vi "放射性半衰期.vi"() -> ()   [LabVIEW 2014]
uses:
  <vilib>/Utility/file.llb/Write To Spreadsheet File (DBL).vi
panel:
  out "m":dbl
  out "每个数据的起始时间":u32
  out "是否为本底":bool
  in  "初始计数率":u32=5000 max=2000000
  out "设置：测量步长":dbl
  out "设置：测量时间":dbl
  out "时间缓存数组":dbl[](array[numeric])
  out "计数缓存数组":dbl[](array[numeric])
  out "图像缓存数组":dbl[][](array[numeric])
  out "n":dbl
  out "现在时间":u32
  in  "按钮_提示":bool caption="提示"
  in  "单道道宽":dbl
  in  "单道阈值":dbl
  out "测量状态":bool
  in  "选项卡控件_实验原理":enum32{"选项卡 1", "选项卡 2"}(tab)
  in  "选项卡控件 实验步骤":enum32{"选项卡 1", "选项卡 2"}(tab)
  in  "按钮_设置成本底":bool
  in  "按钮_保存":bool
  in  "时间步长":dbl caption="秒"
  in  "按钮_设置测量时间":bool
  in  "测量时间":dbl caption="秒"
  out "XY图":T1(graph)
  out "单道计数":i32
  out "停止变量":bool
  in  "按钮_退出":bool
  in  "按钮_开始测量":bool
  in  "按钮_停止":bool
  out "退出":bool
  # "实验：放射性半衰期"
  # "实验仪器"
  # "实验原理"
  # "实验步骤"
  # "操作面板"
  # "1.连接好仪器，放置活性化样品116mIn；\n      2.设置测量时间和测量时间步长；\n      3.点击开始测量，观察计数随着时间增加有着怎样的变化规律，图中的每个点代表每个步长时间间隔内的总计数；\n      4.当测量完成后，点击保存，选择路径并输入文件名；\n      5.点击设置成本底，测量本底10分钟；"
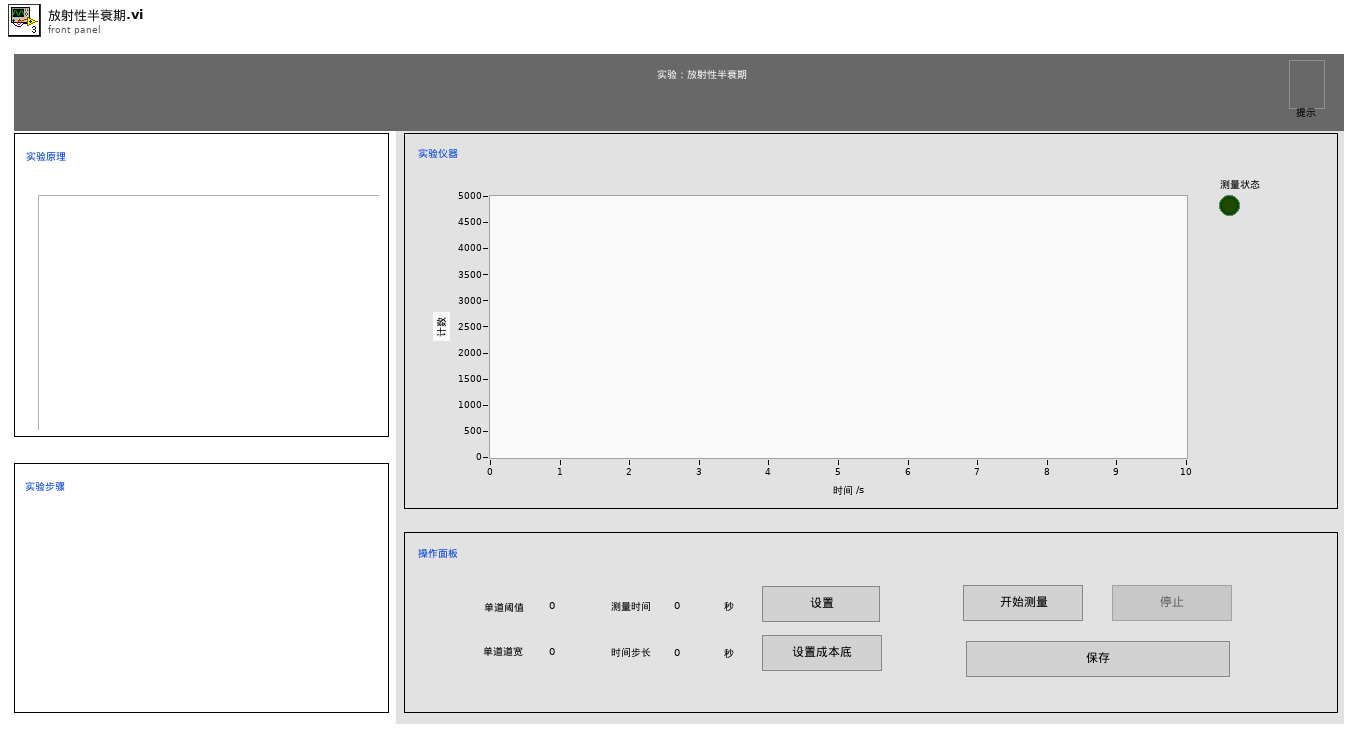
[diagram p1: front panel]
types:
  T1 = cluster{"表一：峰位——能量关系曲线图":cluster{"String":dbl, "String":dbl}[]}[]
  T2 = enum8{"Enabled", "Disabled", "Disabled and Grayed Out"}
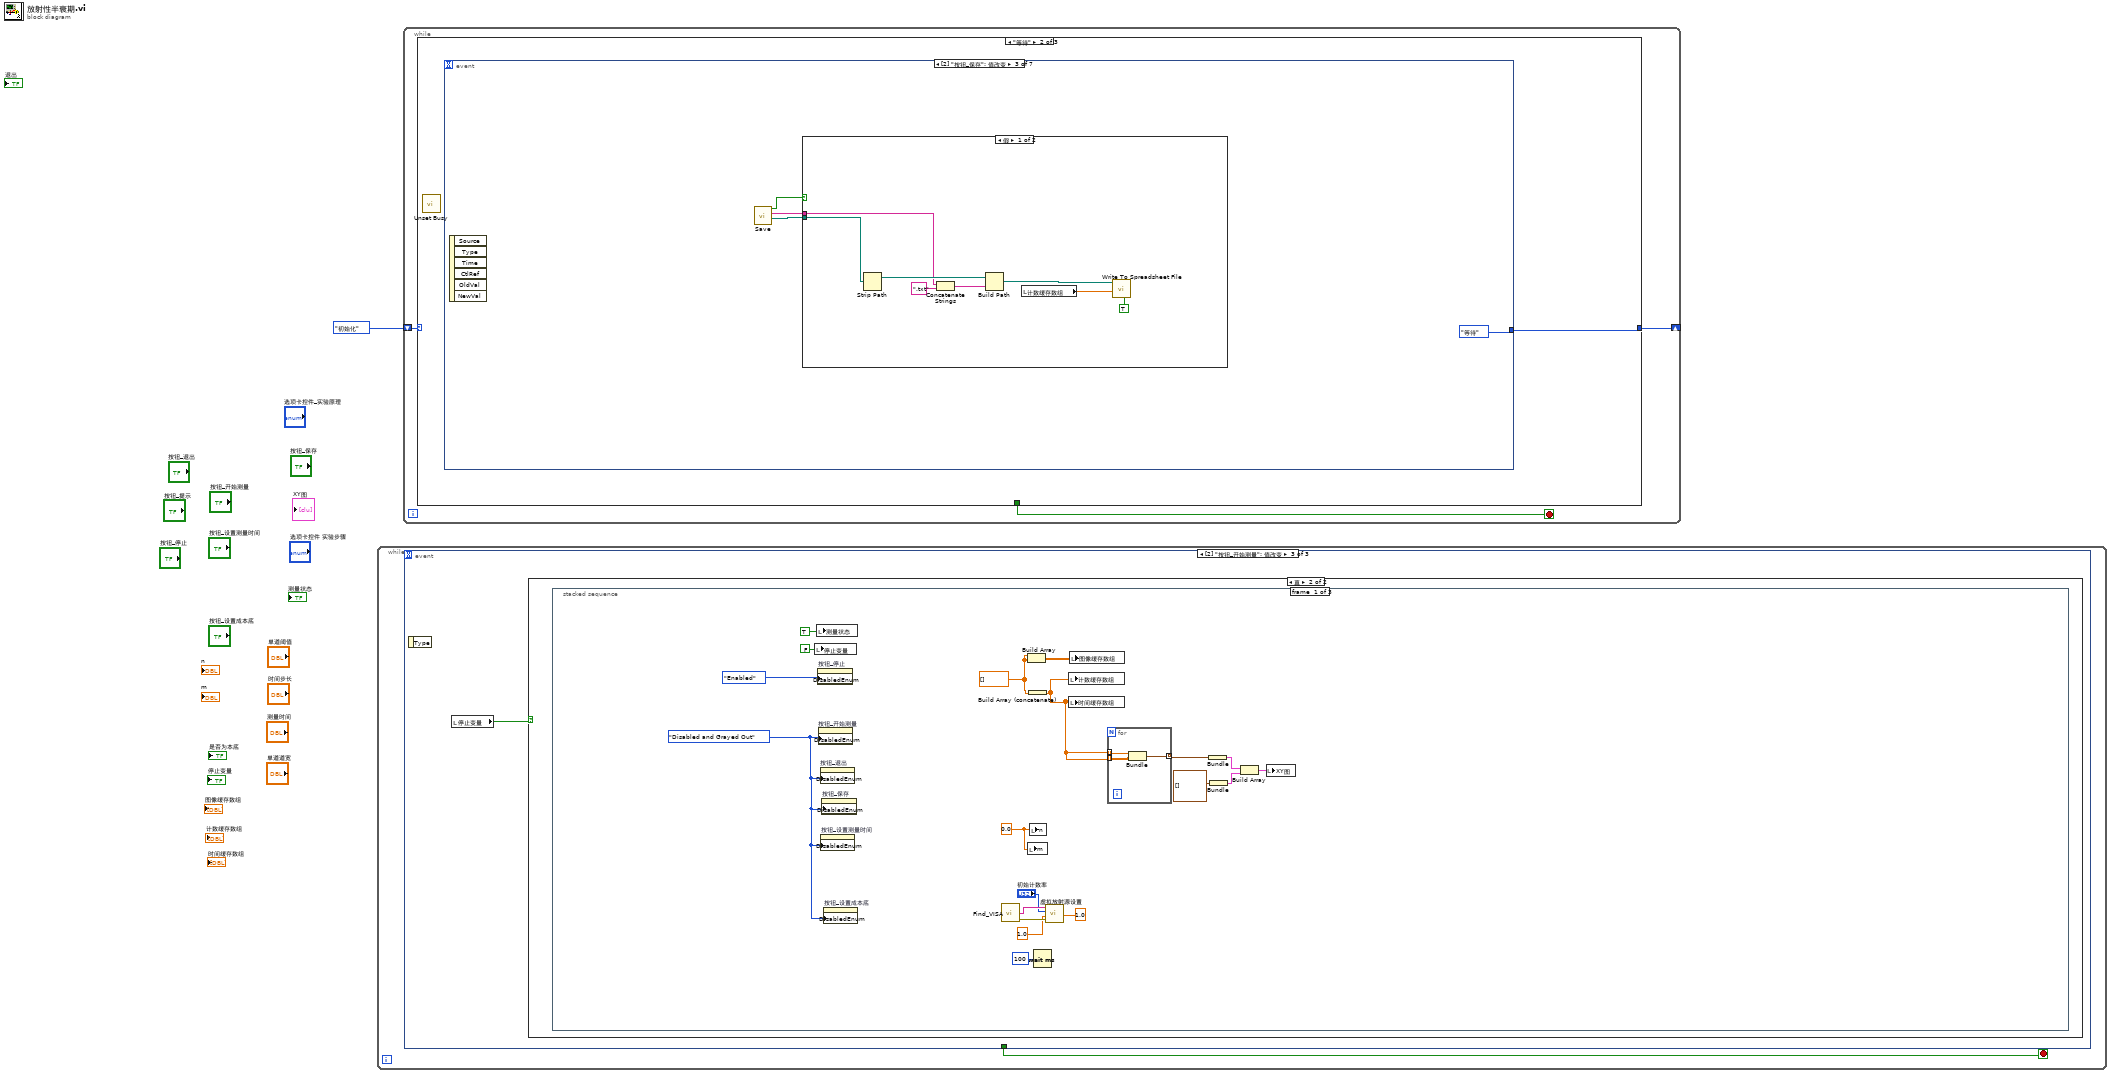
[diagram p0: block diagram]
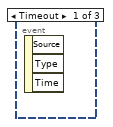
[diagram p2: hidden frame]
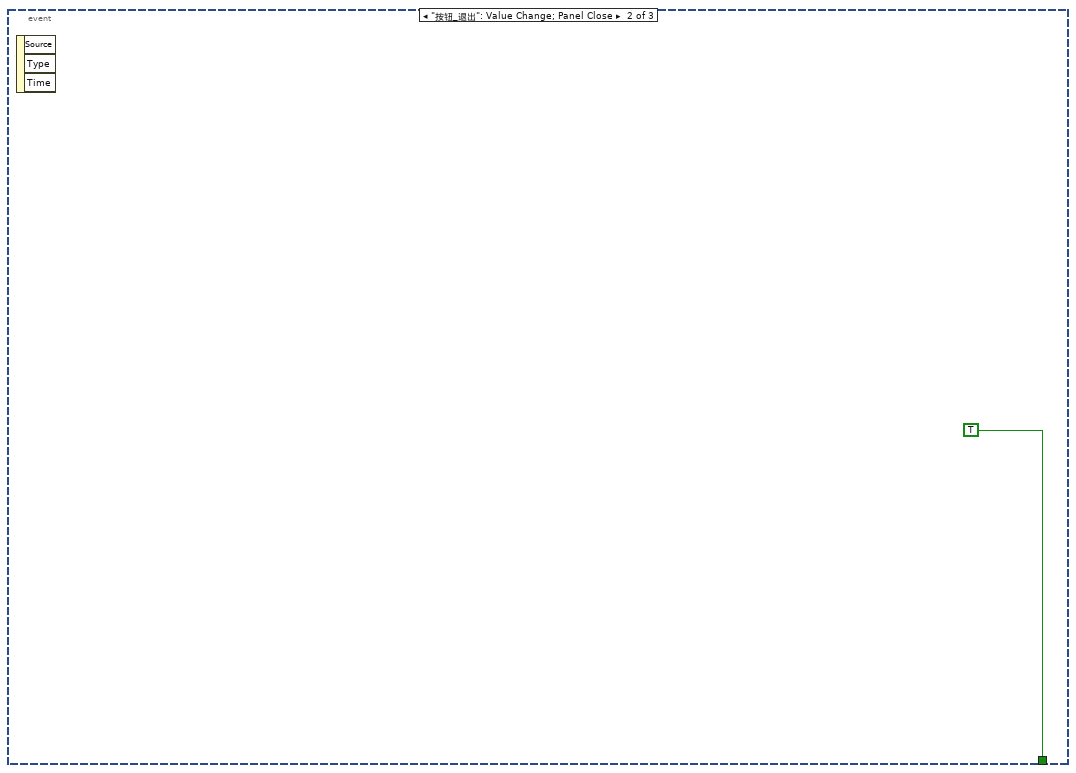
[diagram p3: hidden frame]
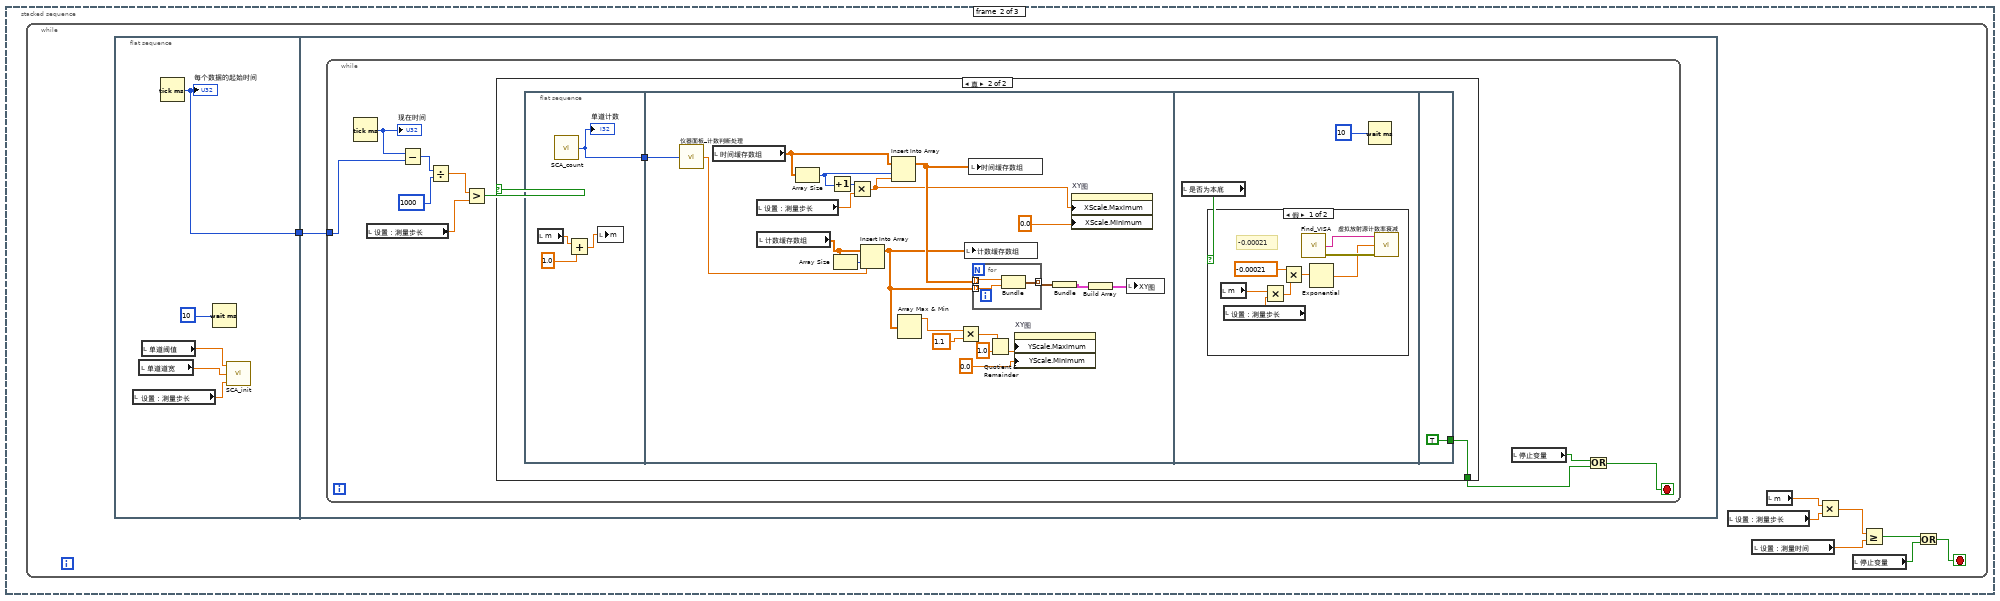
[diagram p5: hidden frame]
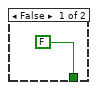
[diagram p6: hidden frame]
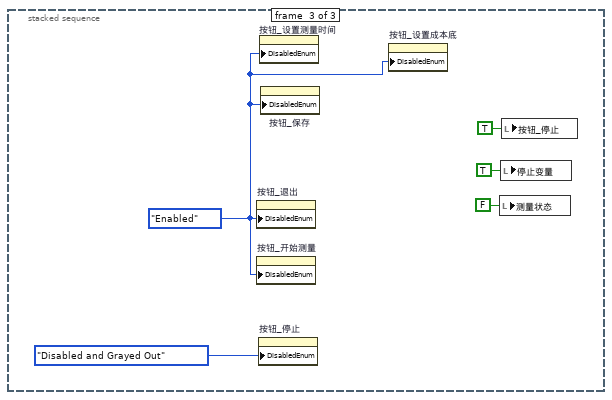
[diagram p8: hidden frame]
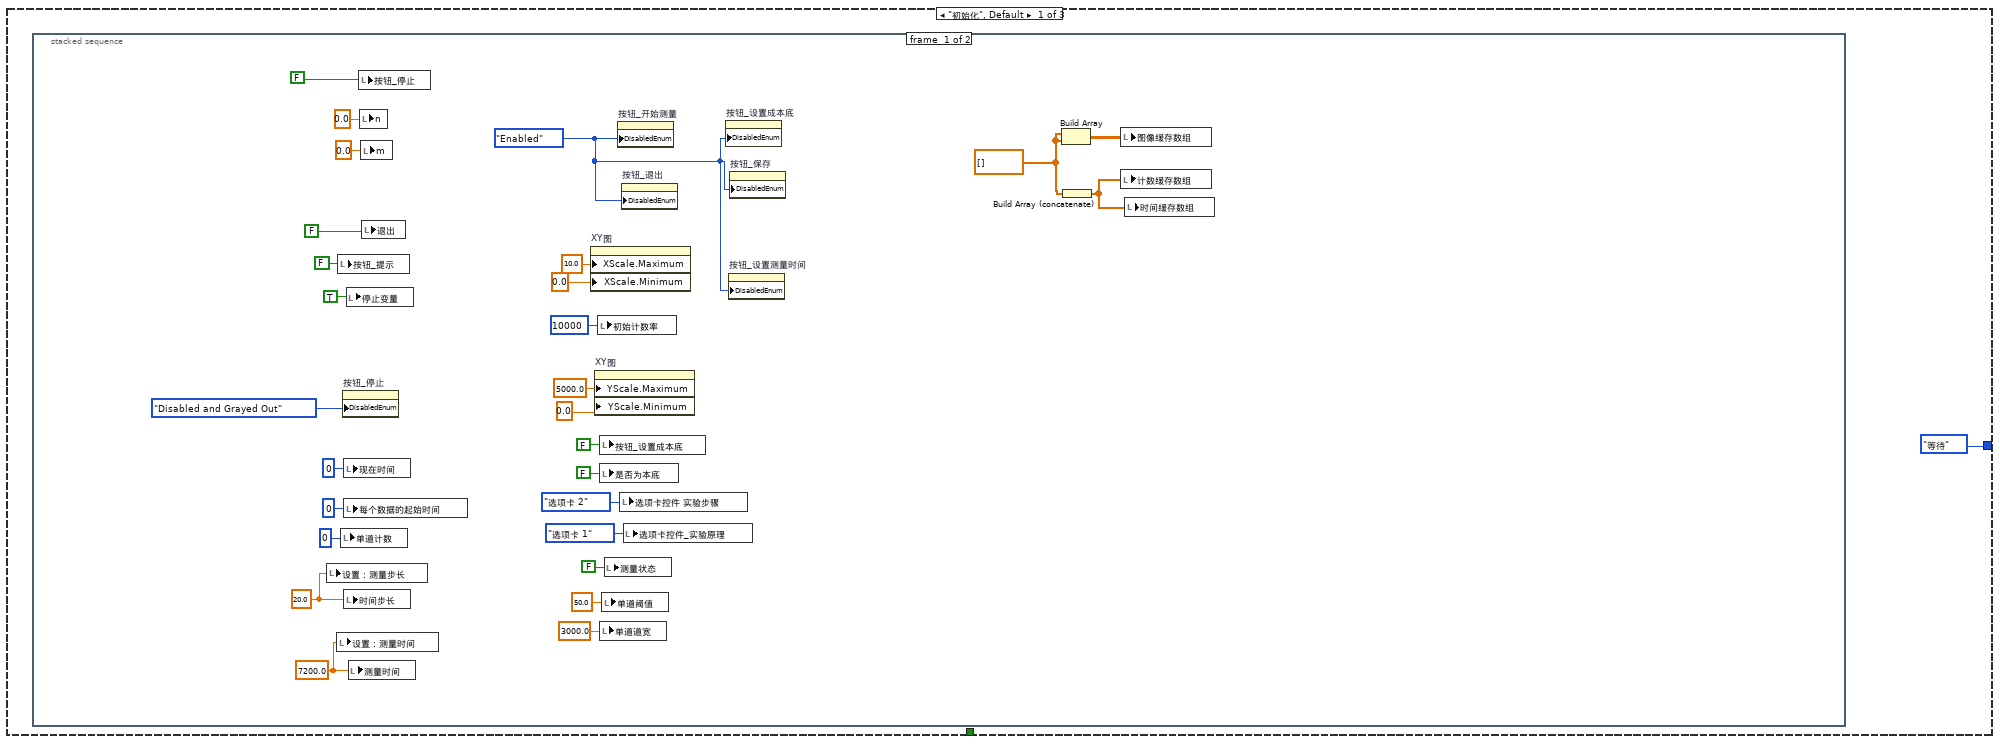
[diagram p9: hidden frame]
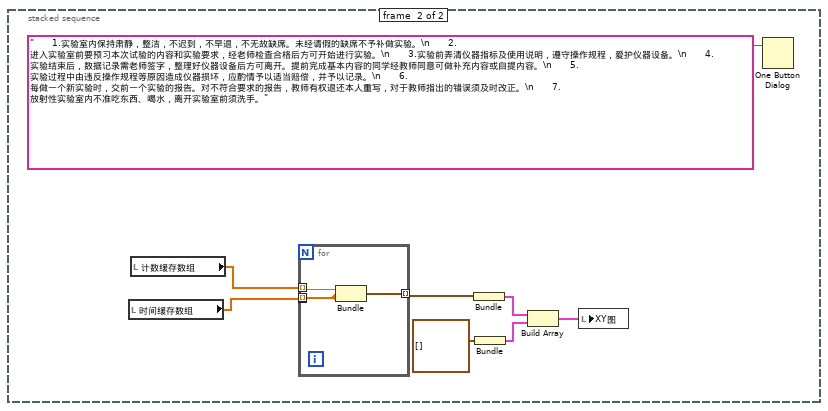
[diagram p10: hidden frame]
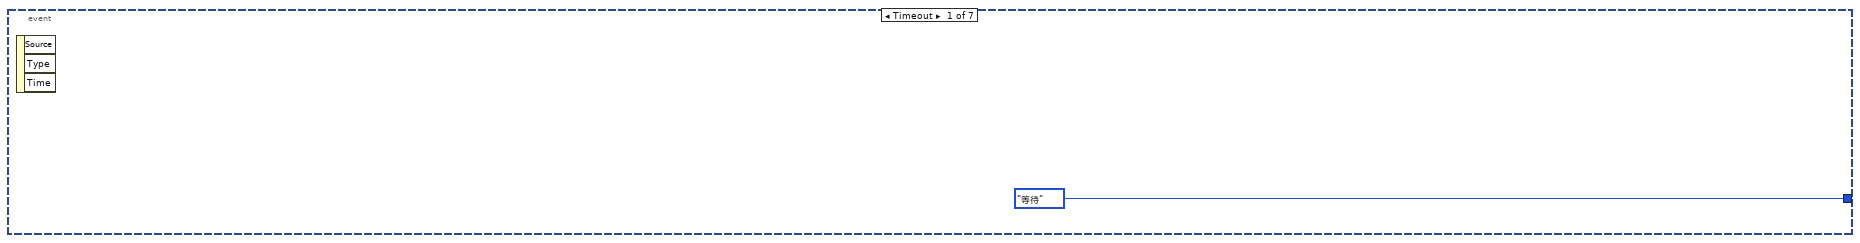
[diagram p11: hidden frame]
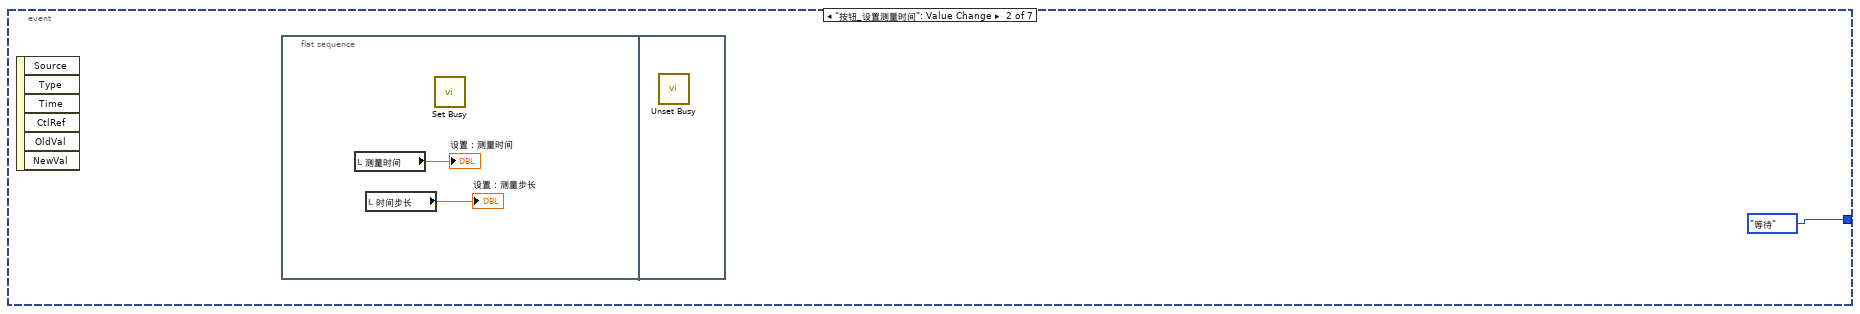
[diagram p12: hidden frame]
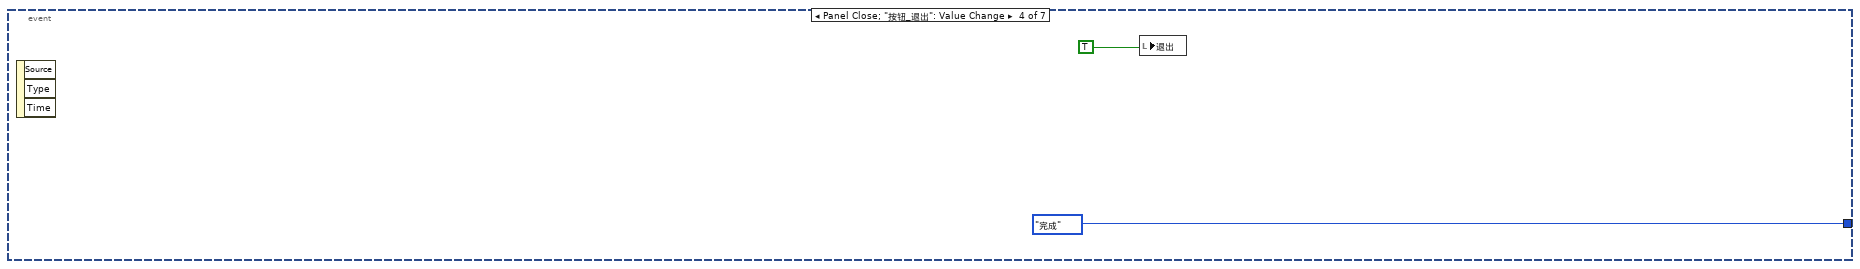
[diagram p14: hidden frame]
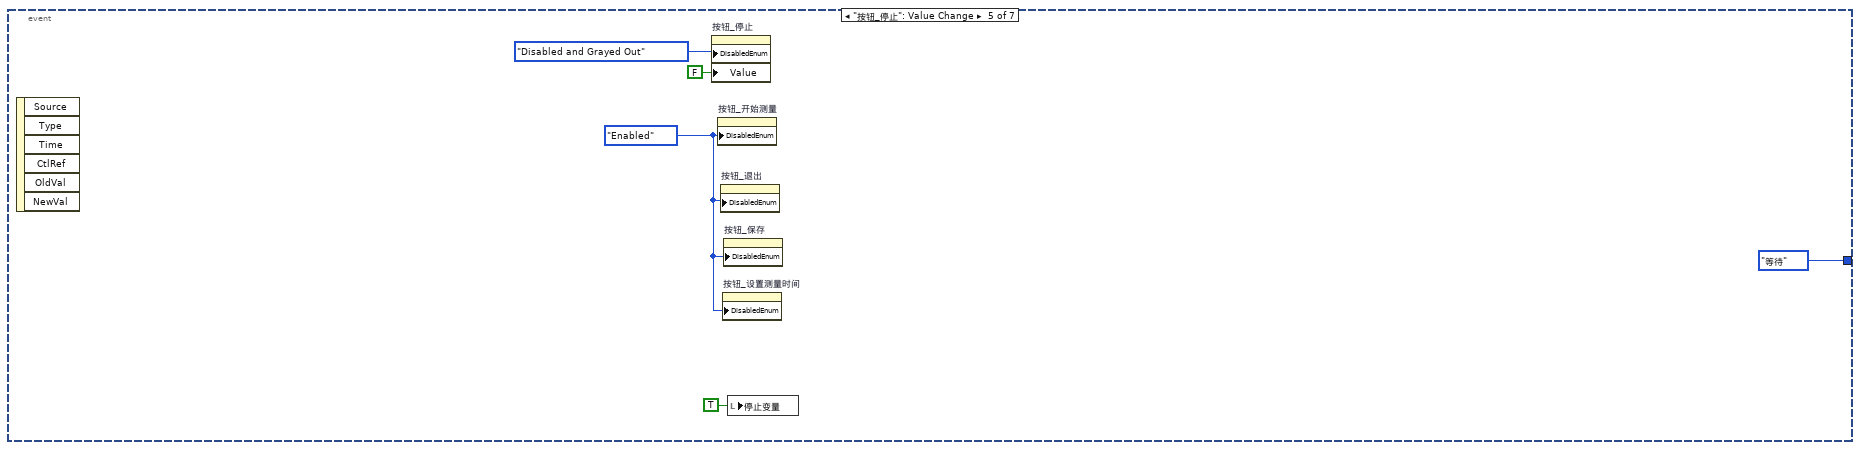
[diagram p15: hidden frame]
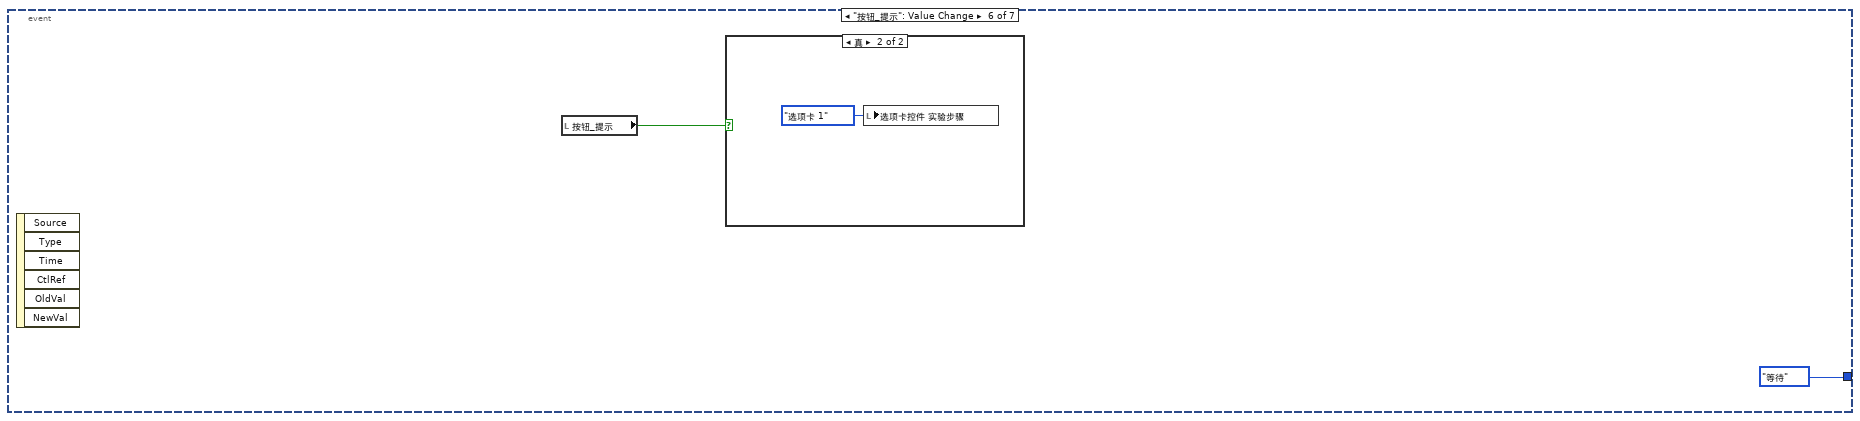
[diagram p16: hidden frame]
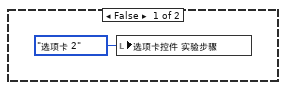
[diagram p17: hidden frame]
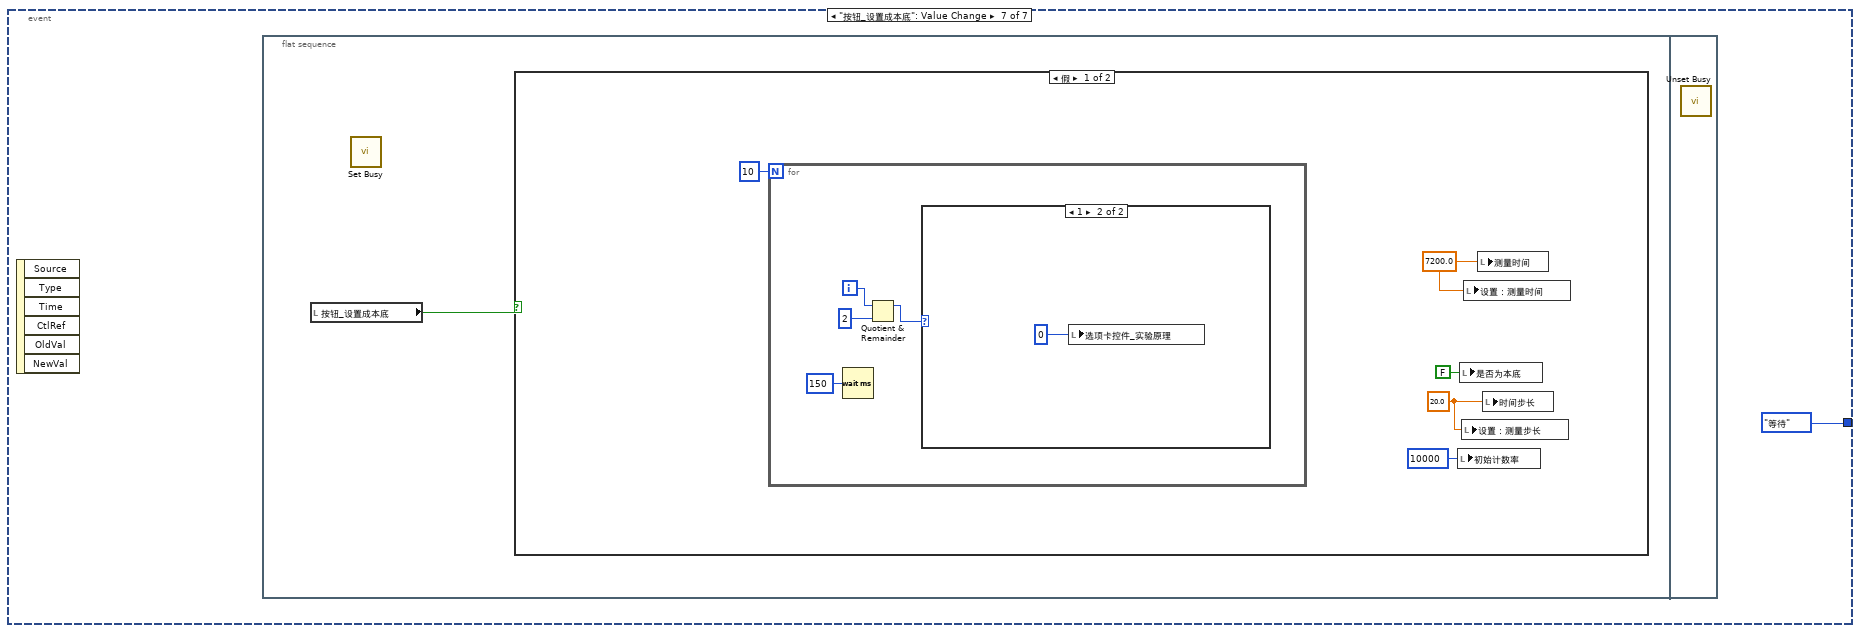
[diagram p18: hidden frame]
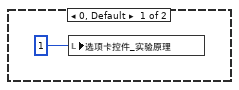
[diagram p19: hidden frame]
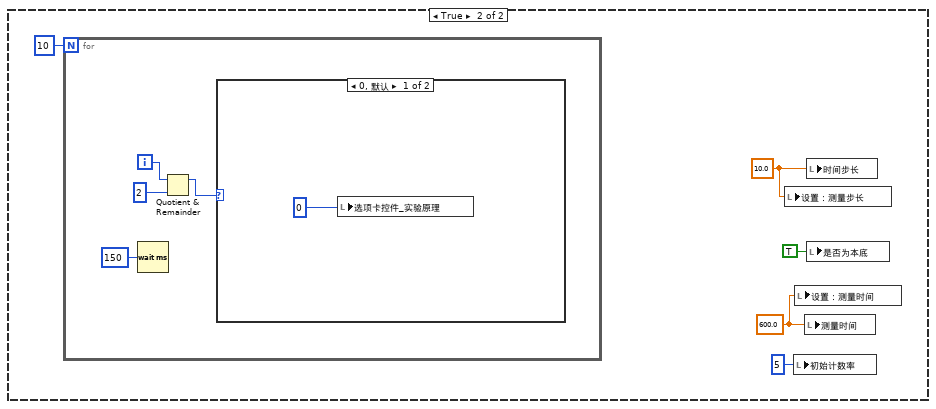
[diagram p20: hidden frame]
diagram:
  n1 = while {
    stop <- w2 stop-if-true
    n2 = event shown="[2] \"按钮_开始测量\": 值改变" {
      selector: _ -> [_ _ _]
      dyn-events: _ -> [_ _ _]
      timeout: _ -> [_ _ _]
      tunnel: [_ TRUE ("高压开关") _] -> w2
      event Timeout {
        n3 = event-data() -> ()  [unwired: 1 in, 3 out]
      }
      event "按钮_退出": Value Change; Panel Close {
        n4 = event-data() -> ()  [unwired: 1 in, 3 out]
      }
      event "按钮_开始测量": Value Change {
        n5 = event-data() -> ()  [unwired: 1 in, 1 out]
        n6 = local read "停止变量"() -> (w4:bool)
        n7 = case shown="真" w4 {
          frame False {
          }
          frame True {
            n8 = stacked-sequence {
              frame #0 {
                w13 = dbl[] []
                w15 = 0.0 ("n")
                w12 = T2."Disabled and Grayed Out" ("禁用")
                n9 = local write "停止变量"(FALSE ("停止变量")) -> ()
                n10 = local write "测量状态"(TRUE ("测量状态")) -> ()
                n11 = property on="按钮_停止" class="Bool (严格)"("DisabledEnum"=T2."Enabled" ("禁用")) -> ()  [unwired: 2 in, 2 out]
                n12 = property on="按钮_开始测量" class="Bool (严格)"("DisabledEnum"=w12) -> ()  [unwired: 2 in, 2 out]
                n13 = property on="按钮_退出" class="Bool (严格)"("DisabledEnum"=w12) -> ()  [unwired: 2 in, 2 out]
                n14 = property on="按钮_设置测量时间" class="Bool (严格)"("DisabledEnum"=w12) -> ()  [unwired: 2 in, 2 out]
                n15 = property on="按钮_保存" class="Bool (严格)"("DisabledEnum"=w12) -> ()  [unwired: 2 in, 2 out]
                n16 = property on="按钮_设置成本底" class="Bool (严格)"("DisabledEnum"=w12) -> ()  [unwired: 2 in, 2 out]
                n17 = call "Find_VISA.vi"() -> ("错误输出"=w10:errorcluster, "虚拟放射源VISA"=w11:string)  [unwired: 3 in, 1 out]
                n18 = Build Array(w13, w13) -> (w22:dbl[][])
                n19 = local write "m"(w15) -> ()
                n20 = Build Array (concatenate)(w13) -> (w17:dbl[])
                n21 = local write "n"(w15) -> ()
                n22 = Wait (ms)(milliseconds to wait=u32 100 ("等待时间（毫秒）")) -> ()  [unwired: 1 out]
                n23 = call "虚拟放射源设置.vi"("放大倍数"=1.0, "错误输入（无错误）"=w10, "最小时间间隔"=1.0 ("衰减"), "计数率"="初始计数率", "VISA资源名称"=w11) -> ()  [unwired: 1 in, 2 out]
                n24 = local write "计数缓存数组"(w17) -> ()
                n25 = local write "时间缓存数组"(w17) -> ()
                n26 = local write "图像缓存数组"(w22) -> ()
                n27 = for {
                  tunnel: w17 -> [w26] mode=indexing
                  tunnel: [w25] -> w19 mode=indexing
                  tunnel: w17 -> [w24] mode=indexing
                  tunnel: [w24] -> _ mode=indexing
                  n28 = Bundle("元素"=w26, "元素"=w24) -> (w25:cluster{"元素":dbl, "元素":dbl})  [unwired: 1 in]
                }
                n29 = Bundle(w19) -> (w20:cluster{cluster{"元素":dbl, "元素":dbl}[]})  [unwired: 1 in]
                n30 = Bundle(cluster{dbl, dbl}[] []) -> (w21:cluster{cluster{dbl, dbl}[]})  [unwired: 1 in]
                n31 = Build Array(w20, w21) -> (w16:cluster{cluster{"元素":dbl, "元素":dbl}[]}[])
                n32 = local write "XY图"(w16) -> ()
              }
              frame #1 {
                n33 = while {
                  stop <- w32 stop-if-true
                  n34 = flat-sequence {
                    tunnel: [w38] -> w31
                    tunnel: w31 -> [w40]
                    frame #0 {
                      n35 = local read "设置：测量步长"() -> (w39:dbl)
                      n36 = local read "单道道宽"() -> (w35:dbl)
                      n37 = local read "单道阈值"() -> (w36:dbl)
                      n38 = Tick Count (ms)() -> (millisecond timer value=w38:u32)
                      "每个数据的起始时间" <- w38
                      n39 = Wait (ms)(milliseconds to wait=u32 10 ("毫秒计时值")) -> ()  [unwired: 1 out]
                      n40 = call "SCA_init.vi"("runtime(秒)"=w39, "单道1道宽"=w35, "单道1阈值电压"=w36) -> ()
                    }
                    frame #1 {
                      n41 = while {
                        tunnel: w40 -> [w45]
                        stop <- w41 stop-if-true
                        n42 = Tick Count (ms)() -> (millisecond timer value=w44:u32)
                        "现在时间" <- w44
                        n43 = local read "设置：测量步长"() -> (w49:dbl)
                        n44 = Subtract(x=w44, y=w45) -> (x-y=w46:u32)
                        n45 = Divide(x=w46, y=1000) -> (x/y=w47:dbl)
                        n46 = Greater?(x=w47, y=w49) -> (0:w50:bool)
                        n47 = case shown="真" w50 {
                          tunnel: [FALSE w52] -> w42
                          frame False {
                          }
                          frame True {
                            n48 = flat-sequence {
                              tunnel: [w57] -> w53
                              tunnel: w53 -> [w58]
                              tunnel: [TRUE] -> w52
                              frame #0 {
                                n49 = local read "m"() -> (w56:dbl)
                                n50 = call "SCA_count.vi"() -> ("Acnt"=w57:i32)
                                "单道计数" <- w57
                                n51 = Add(x=w56, y=1.0) -> (x+y=w54:dbl)
                                n52 = local write "m"(w54) -> ()
                              }
                              frame #1 {
                                n53 = call "仪器面板_计数判断处理.vi"("数值"=w58) -> ("数值 2"=w67:dbl)
                                n54 = local read "时间缓存数组"() -> (w73:dbl[])
                                n55 = local read "设置：测量步长"() -> (w69:dbl)
                                n56 = local read "计数缓存数组"() -> (w71:dbl[])
                                n57 = Array Size(array=w73) -> (size(s)=w68:i32)
                                n58 = Increment(x=w68) -> (x+1=w70:i32)
                                n59 = Array Size(array=w71) -> (size(s)=w72:i32)
                                n60 = Multiply(x=w70, y=w69) -> (x*y=w59:dbl)
                                n61 = Insert Into Array(array=w71, index=w72, new element=w67) -> (w66:dbl[])
                                n62 = Insert Into Array(array=w73, index=w68, new element=w59) -> (w74:dbl[])
                                n63 = Array Max & Min(array=w66) -> (max value=w62:dbl)  [unwired: 3 out]
                                n64 = Multiply(x=w62, y=1.1) -> (x*y=w64:dbl)
                                n65 = local write "计数缓存数组"(w66) -> ()
                                n66 = local write "时间缓存数组"(w74) -> ()
                                n67 = for {
                                tunnel: w74 -> [w81] mode=indexing
                                tunnel: [w80] -> w77 mode=indexing
                                tunnel: w66 -> [w79] mode=indexing
                                n68 = Bundle(w81, w79) -> (w80:cluster{dbl, dbl})  [unwired: 1 in]
                                }
                                n69 = Quotient & Remainder(x=w64, y=1.0) -> (floor(x/y)=w60:dbl)  [unwired: 1 out]
                                n70 = property on="XY图" class="XYGraph (严格)"("YScale.Maximum"=w60, "YScale.Minimum"=0.0 ("X标尺.范围:最小值")) -> ()  [unwired: 2 in, 2 out]
                                n71 = Bundle(w77) -> (w78:cluster{cluster{dbl, dbl}[]})  [unwired: 1 in]
                                n72 = property on="XY图" class="XYGraph (严格)"("XScale.Maximum"=w59, "XScale.Minimum"=0.0 ("X标尺.范围:最小值")) -> ()  [unwired: 2 in, 2 out]
                                n73 = Build Array(w78) -> (w76:cluster{cluster{dbl, dbl}[]}[])
                                n74 = local write "XY图"(w76) -> ()
                              }
                              frame #2 {
                                n75 = local read "是否为本底"() -> (w82:bool)
                                n76 = case shown="假" w82 {
                                frame False {
                                # "-0.00021"
                                n77 = local read "m"() -> (w85:dbl)
                                n78 = local read "设置：测量步长"() -> (w84:dbl)
                                n79 = Multiply(x=w85, y=w84) -> (x*y=w86:dbl)
                                n80 = Multiply(x=-0.00021, y=w86) -> (x*y=w87:dbl)
                                n81 = call "Find_VISA.vi"() -> ("错误输出"=w91:errorcluster, "虚拟放射源VISA"=w89:string)  [unwired: 3 in, 1 out]
                                n82 = Exponential(1:w87) -> (0:w90:dbl)
                                n83 = call "虚拟放射源计数率衰减.vi"("错误输入（无错误）"=w91, "衰减"=w90, "VISA资源名称"=w89) -> ()  [unwired: 2 out]
                                }
                                frame True {
                                }
                                }
                                n84 = Wait (ms)(milliseconds to wait=u32 10 ("毫秒计时值")) -> ()  [unwired: 1 out]
                              }
                              frame #3 {
                              }
                            }
                          }
                        }
                        n85 = local read "停止变量"() -> (w43:bool)
                        n86 = Or(x=w43, y=w42) -> (x .or. y?=w41:bool)
                      }
                    }
                  }
                  n87 = local read "设置：测量步长"() -> (w29:dbl)
                  n88 = local read "设置：测量时间"() -> (w27:dbl)
                  n89 = local read "m"() -> (w30:dbl)
                  n90 = Multiply(x=w30, y=w29) -> (x*y=w28:dbl)
                  n91 = local read "停止变量"() -> (w34:bool)
                  n92 = Greater Or Equal?(x=w28, y=w27) -> (x >= y?=w33:bool)
                  n93 = Or(x=w33, y=w34) -> (x .or. y?=w32:bool)
                }
              }
              frame #2 {
                w95 = T2."Enabled" ("禁用")
                n94 = property on="按钮_退出" class="Bool (严格)"("DisabledEnum"=w95) -> ()  [unwired: 2 in, 2 out]
                n95 = property on="按钮_开始测量" class="Bool (严格)"("DisabledEnum"=w95) -> ()  [unwired: 2 in, 2 out]
                n96 = property on="按钮_停止" class="Bool (严格)"("DisabledEnum"=T2."Disabled and Grayed Out" ("禁用")) -> ()  [unwired: 2 in, 2 out]
                n97 = property on="按钮_设置测量时间" class="Bool (严格)"("DisabledEnum"=w95) -> ()  [unwired: 2 in, 2 out]
                n98 = property on="按钮_保存" class="Bool (严格)"("DisabledEnum"=w95) -> ()  [unwired: 2 in, 2 out]
                n99 = property on="按钮_设置成本底" class="Bool (严格)"("DisabledEnum"=w95) -> ()  [unwired: 2 in, 2 out]
                n100 = local write "测量状态"(FALSE ("测量状态")) -> ()
                n101 = local write "停止变量"(TRUE ("停止变量")) -> ()
                n102 = local write "按钮_停止"(TRUE ("按钮_停止")) -> ()
              }
            }
          }
        }
      }
    }
  }
  n103 = while {
    shift-right: [w99] -> _
    shift-left: enum16{"初始化", "等待", "完成"}."初始化" -> [w100]
    stop <- w98 stop-if-true
    n104 = case shown="\"等待\"" w100 {
      tunnel: [enum16{"初始化", "等待", "完成"}."等待" w141 enum16{"初始化", "等待", "完成"}."完成"] -> w99
      tunnel: [_ _ TRUE] -> w98
      frame "初始化", Default {
        n105 = stacked-sequence {
          frame #0 {
            w113 = dbl[] []
            w119 = 7200.0 ("测量时间设置")
            w120 = 20.0 ("设置测量时间步长")
            w110 = T2."Enabled" ("禁用")
            n106 = local write "设置：测量步长"(w120) -> ()
            n107 = local write "设置：测量时间"(w119) -> ()
            n108 = local write "按钮_提示"(FALSE ("按钮_提示")) -> ()
            n109 = local write "单道计数"(0 ("单道计数")) -> ()
            n110 = property on="按钮_停止" class="Bool (严格)"("DisabledEnum"=T2."Disabled and Grayed Out" ("禁用")) -> ()  [unwired: 2 in, 2 out]
            n111 = local write "现在时间"(u32 0 ("现在时间")) -> ()
            n112 = local write "每个数据的起始时间"(u32 0 ("每个数据的起始时间")) -> ()
            n113 = local write "时间步长"(w120) -> ()
            n114 = local write "停止变量"(TRUE ("停止变量")) -> ()
            n115 = local write "测量时间"(w119) -> ()
            n116 = local write "按钮_停止"(FALSE ("高压开关")) -> ()
            n117 = local write "n"(0.0 ("n")) -> ()
            n118 = local write "m"(0.0 ("m")) -> ()
            n119 = local write "退出"(FALSE ("高压开关")) -> ()
            n120 = property on="XY图" class="XYGraph (严格)"("XScale.Maximum"=10.0 ("X标尺.范围:最大值"), "XScale.Minimum"=0.0 ("X标尺.范围:最小值")) -> ()  [unwired: 2 in, 2 out]
            n121 = property on="XY图" class="XYGraph (严格)"("YScale.Maximum"=5000.0 ("Y标尺.范围:最大值"), "YScale.Minimum"=0.0 ("Y标尺.范围:最小值")) -> ()  [unwired: 2 in, 2 out]
            n122 = local write "初始计数率"(u32 10000 ("初始计数率")) -> ()
            n123 = local write "按钮_设置成本底"(FALSE ("按钮_设置成本底")) -> ()
            n124 = local write "是否为本底"(FALSE ("是否为本底")) -> ()
            n125 = local write "单道道宽"(3000.0 ("单道道宽")) -> ()
            n126 = local write "单道阈值"(50.0 ("单道阈值")) -> ()
            n127 = local write "测量状态"(FALSE ("测量状态")) -> ()
            n128 = property on="按钮_开始测量" class="Bool (严格)"("DisabledEnum"=w110) -> ()  [unwired: 2 in, 2 out]
            n129 = local write "选项卡控件 实验步骤"(enum32{"选项卡 1", "选项卡 2"}."选项卡 2" ("选项卡控件 实验步骤")) -> ()
            n130 = property on="按钮_退出" class="Bool (严格)"("DisabledEnum"=w110) -> ()  [unwired: 2 in, 2 out]
            n131 = local write "选项卡控件_实验原理"(enum32{"选项卡 1", "选项卡 2"}."选项卡 1" ("选项卡控件_实验原理")) -> ()
            n132 = property on="按钮_设置成本底" class="Bool (严格)"("DisabledEnum"=w110) -> ()  [unwired: 2 in, 2 out]
            n133 = property on="按钮_设置测量时间" class="Bool (严格)"("DisabledEnum"=w110) -> ()  [unwired: 2 in, 2 out]
            n134 = property on="按钮_保存" class="Bool (严格)"("DisabledEnum"=w110) -> ()  [unwired: 2 in, 2 out]
            n135 = Build Array(w113, w113) -> (w117:dbl[][])
            n136 = Build Array (concatenate)(w113) -> (w116:dbl[])
            n137 = local write "图像缓存数组"(w117) -> ()
            n138 = local write "计数缓存数组"(w116) -> ()
            n139 = local write "时间缓存数组"(w116) -> ()
          }
          frame #1 {
            n140 = local read "时间缓存数组"() -> (w131:dbl[])
            n141 = local read "计数缓存数组"() -> (w132:dbl[])
            n142 = for {
              tunnel: w132 -> [w140] mode=indexing
              tunnel: [w139] -> w134 mode=indexing
              tunnel: w131 -> [w138] mode=indexing
              tunnel: [w138] -> _ mode=indexing
              n143 = Bundle(w140, w138) -> (w139:cluster{dbl, dbl})  [unwired: 1 in]
            }
            n144 = Bundle(w134) -> (w135:cluster{cluster{dbl, dbl}[]})  [unwired: 1 in]
            n145 = Bundle(cluster{dbl, dbl}[] []) -> (w136:cluster{cluster{dbl, dbl}[]})  [unwired: 1 in]
            n146 = Build Array(w135, w136) -> (w130:cluster{cluster{dbl, dbl}[]}[])
            n147 = local write "XY图"(w130) -> ()
            n148 = One Button Dialog(message="      1.实验室内保持肃静，整洁，不迟到，不早退，不无故缺席。未经请假的缺席不予补做实验。\n      2.进入实验室前要预习本次试验的内容和实验要求，经老师检查合格后方可开始进行实验。\n      3.实验前弄清仪器指标及使用说明，遵守操作规程，爱护仪器设备。\n      4.实验结束后，数据记录需老师签字，整理好仪器设备后方可离开。提前完成基本内容的同学经教师同意可做补充内容或自提内容。\n      5.实验过程中由违反操作规程等原因造成仪器损坏，应酌情予以适当赔偿，并予以记录。\n      6.每做一个新实验时，交前一个实验的报告。对不符合要求的报告，教师有权退还本人重写，对于教师指出的错误须及时改正。\n      7.放射性实验室内不准吃东西、喝水，离开实验室前须洗手。" ("消息")) -> ()  [unwired: 1 in, 1 out]
          }
        }
      }
      frame "等待" {
        n149 = call <vilib>:"Unset Busy.vi"() -> ()  [unwired: 11 in, 1 out]
        n150 = event shown="[2] \"按钮_保存\": 值改变" {
          selector: _ -> [_ _ _ _ _ _ _]
          dyn-events: _ -> [_ _ _ _ _ _ _]
          timeout: _ -> [_ _ _ _ _ _ _]
          tunnel: [enum16{"初始化", "等待", "完成"}."等待" enum16{"初始化", "等待", "完成"}."等待" enum16{"初始化", "等待", "完成"}."等待" enum16{"初始化", "等待", "完成"}."完成" enum16{"初始化", "等待", "完成"}."等待" enum16{"初始化", "等待", "完成"}."等待" enum16{"初始化", "等待", "完成"}."等待"] -> w141
          event Timeout {
            n151 = event-data() -> ()  [unwired: 1 in, 3 out]
          }
          event "按钮_设置测量时间": Value Change {
            n152 = event-data() -> ()  [unwired: 1 in, 6 out]
            n153 = flat-sequence {
              frame #0 {
                n154 = local read "测量时间"() -> (→"设置：测量时间":dbl)
                n155 = local read "时间步长"() -> (→"设置：测量步长":dbl)
                n156 = call <vilib>:"Set Busy.vi"() -> ()  [unwired: 10 in, 2 out]
              }
              frame #1 {
                n157 = call <vilib>:"Unset Busy.vi"() -> ()  [unwired: 11 in, 1 out]
              }
            }
          }
          event "按钮_保存": Value Change {
            n158 = event-data() -> ()  [unwired: 1 in, 6 out]
            n159 = call "Save.vi"() -> ("保存数据文件至： 2"=w147:path, "数据文件名称： 2"=w148:string, "是否取消？"=w146:bool)  [unwired: 9 in]
            n160 = case shown="假" w146 {
              tunnel: w148 -> [w151 _]
              tunnel: w147 -> [w150 _]
              frame False {
                n161 = Strip Path(path=w150) -> (stripped path=w155:path)  [unwired: 1 out]
                n162 = Concatenate Strings(w151, ".txt" ("字符串")) -> (w154:string)
                n163 = Build Path(base path=w155, name or relative path=w154) -> (appended path=w156:path)
                n164 = local read "计数缓存数组"() -> (w157:dbl[])
                n165 = call-poly <vilib>:"Write To Spreadsheet File.vi"("transpose? (no:F)"=TRUE, "1D data"=w157, "file path (dialog if empty)"=w156) -> ()  [unwired: 5 in, 1 out]
              }
              frame True {
              }
            }
          }
          event Panel Close; "按钮_退出": Value Change {
            n166 = event-data() -> ()  [unwired: 1 in, 3 out]
            n167 = local write "退出"(TRUE ("高压开关")) -> ()
          }
          event "按钮_停止": Value Change {
            w161 = T2."Enabled" ("禁用")
            n168 = event-data() -> ()  [unwired: 1 in, 6 out]
            n169 = property on="按钮_停止" class="Bool (严格)"("DisabledEnum"=T2."Disabled and Grayed Out" ("禁用"), "Value"=FALSE ("按钮_停止")) -> ()  [unwired: 2 in, 2 out]
            n170 = property on="按钮_开始测量" class="Bool (严格)"("DisabledEnum"=w161) -> ()  [unwired: 2 in, 2 out]
            n171 = property on="按钮_退出" class="Bool (严格)"("DisabledEnum"=w161) -> ()  [unwired: 2 in, 2 out]
            n172 = property on="按钮_设置测量时间" class="Bool (严格)"("DisabledEnum"=w161) -> ()  [unwired: 2 in, 2 out]
            n173 = property on="按钮_保存" class="Bool (严格)"("DisabledEnum"=w161) -> ()  [unwired: 2 in, 2 out]
            n174 = local write "停止变量"(TRUE ("停止变量")) -> ()
          }
          event "按钮_提示": Value Change {
            n175 = event-data() -> ()  [unwired: 1 in, 6 out]
            n176 = local read "按钮_提示"() -> (w165:bool)
            n177 = case shown="真" w165 {
              frame False {
                n178 = local write "选项卡控件 实验步骤"(enum32{"选项卡 1", "选项卡 2"}."选项卡 2" ("选项卡控件 实验步骤")) -> ()
              }
              frame True {
                n179 = local write "选项卡控件 实验步骤"(enum32{"选项卡 1", "选项卡 2"}."选项卡 1" ("选项卡控件 实验步骤")) -> ()
              }
            }
          }
          event "按钮_设置成本底": Value Change {
            n180 = event-data() -> ()  [unwired: 1 in, 6 out]
            n181 = flat-sequence {
              frame #0 {
                n182 = local read "按钮_设置成本底"() -> (w170:bool)
                n183 = call <vilib>:"Set Busy.vi"() -> ()  [unwired: 10 in, 2 out]
                n184 = case shown="假" w170 {
                  frame False {
                    w172 = 7200.0 ("测量时间设置")
                    w171 = 20.0 ("设置测量时间步长")
                    n185 = for {
                      N: 10 -> [_]
                      i -> [w178]
                      n186 = Wait (ms)(milliseconds to wait=u32 150 ("等待时间（毫秒）")) -> ()  [unwired: 1 out]
                      n187 = Quotient & Remainder(x=w178, y=2) -> (x-y*floor(x/y)=w179:i32)  [unwired: 1 out]
                      n188 = case shown="1" w179 {
                        frame 0, Default {
                          n189 = local write "选项卡控件_实验原理"(1) -> ()
                        }
                        frame 1 {
                          n190 = local write "选项卡控件_实验原理"(0) -> ()
                        }
                      }
                    }
                    n191 = local write "初始计数率"(u32 10000 ("初始计数率")) -> ()
                    n192 = local write "是否为本底"(FALSE ("是否为本底")) -> ()
                    n193 = local write "设置：测量步长"(w171) -> ()
                    n194 = local write "设置：测量时间"(w172) -> ()
                    n195 = local write "测量时间"(w172) -> ()
                    n196 = local write "时间步长"(w171) -> ()
                  }
                  frame True {
                    w182 = 600.0 ("测量时间设置")
                    w183 = 10.0 ("设置测量时间步长")
                    n197 = for {
                      N: 10 -> [_]
                      i -> [w189]
                      n198 = Wait (ms)(milliseconds to wait=u32 150 ("等待时间（毫秒）")) -> ()  [unwired: 1 out]
                      n199 = Quotient & Remainder(x=w189, y=2) -> (x-y*floor(x/y)=w190:i32)  [unwired: 1 out]
                      n200 = case shown="0, 默认" w190 {
                        frame 0, Default {
                          n201 = local write "选项卡控件_实验原理"(0) -> ()
                        }
                        frame 1 {
                          n202 = local write "选项卡控件_实验原理"(1) -> ()
                        }
                      }
                    }
                    n203 = local write "设置：测量步长"(w183) -> ()
                    n204 = local write "初始计数率"(u32 5 ("初始计数率")) -> ()
                    n205 = local write "设置：测量时间"(w182) -> ()
                    n206 = local write "测量时间"(w182) -> ()
                    n207 = local write "时间步长"(w183) -> ()
                    n208 = local write "是否为本底"(TRUE ("是否为本底")) -> ()
                  }
                }
              }
              frame #1 {
                n209 = call <vilib>:"Unset Busy.vi"() -> ()  [unwired: 11 in, 1 out]
              }
            }
          }
        }
      }
      frame "完成" {
      }
    }
  }
